vi "Query Active DUT Connector Catalog.vi"(8 "error in (no error)":errorcluster, 11 "VISA resource name":refnum<visa-resource-name>) -> (0 "error out":errorcluster, 2 "Connectors":string, 3 "VISA resource name out":refnum<visa-resource-name>)   [LabVIEW 2015, in "Rohde&Schwarz CMXP Base.lvlib"]
doc: "Queries a list of all antenna connectors of the active DUT.\n\nAttribute:\nRSCMXPBASE_ATTR_ACTIVE_DUT_CONNECTOR_CATALOG\n\nRemote-control command:\nCATalog:DUT:CONNector?"
uses:
  <instrlib>/Rohde&Schwarz CMXP Base/Rohde&Schwarz CMXP Base.lvlib
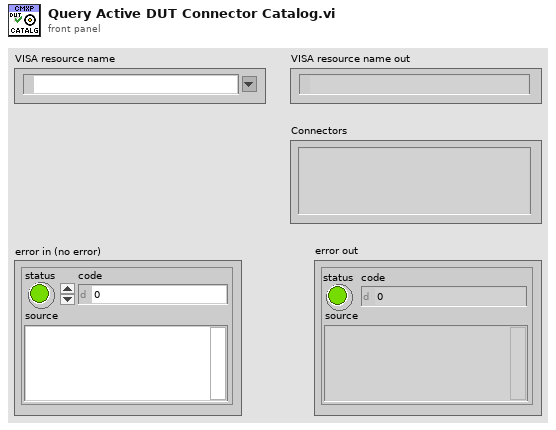
[diagram p1: front panel]
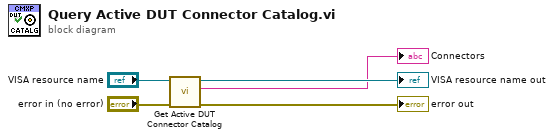
[diagram p0: block diagram]
diagram:
  n1 = call "Get Active DUT Connector Catalog"("error in (no error)"="error in (no error)", "instrument handle"="VISA resource name") -> ("error out"=→"error out":errorcluster, "Active DUT Connector Catalog"=→"Connectors":string, "instrument handle out"=→"VISA resource name out":refnum<visa-resource-name>)  [unwired: 7 in]
